vi "SN_core_parser.vi"(9 "SN in":string, 11 "regular expression":string) -> (1 "SN status":enum16{"SN PASS", "SN FAIL"}(ring), 3 "match?":bool)   [LabVIEW 2024]
panel:
  # "lit when match"
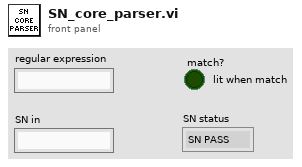
[diagram p1: front panel]
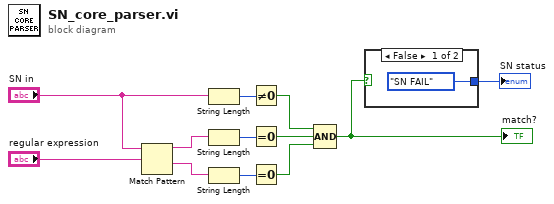
[diagram p0: block diagram]
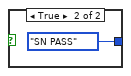
[diagram p2: hidden frame]
diagram:
  n1 = Match Pattern(string="SN in", regular expression="regular expression") -> (before substring=w3:string, after substring=w4:string)  [unwired: 1 in, 2 out]
  n2 = String Length(string="SN in") -> (length=w7:i32)
  n3 = String Length(string=w3) -> (length=w5:i32)
  n4 = String Length(string=w4) -> (length=w6:i32)
  n5 = Not Equal To 0?(x=w7) -> (x != 0?=w10:bool)
  n6 = Equal To 0?(x=w5) -> (x = 0?=w9:bool)
  n7 = Equal To 0?(x=w6) -> (x = 0?=w8:bool)
  n8 = Compound Arithmetic op=AND(w10, w9, w8) -> (w2:bool)
  "match?" <- w2
  n9 = case shown="False" w2 {
    tunnel: [enum16{"SN PASS", "SN FAIL"}."SN FAIL" ("SN status") enum16{"SN PASS", "SN FAIL"}."SN PASS" ("SN status")] -> w1
    frame False {
    }
    frame True {
    }
  }
  "SN status" <- w1
